vi "Get DAQmx Channels Status.vi"(0 "DAQmx task":refnum<k21>, 9 "status info in":variant, 11 "error in":errorcluster) -> (4 "DAQmx task":refnum<k21>, 6 "channel errors":bool, 10 "status info out":variant, 15 "error out":errorcluster)   [LabVIEW 2024, in "DSA_CFG_ACQ.lvlib"]
uses:
  DSA_CFG_ACQ.lvlib
  <resource>/objmgr/daqmx.rc
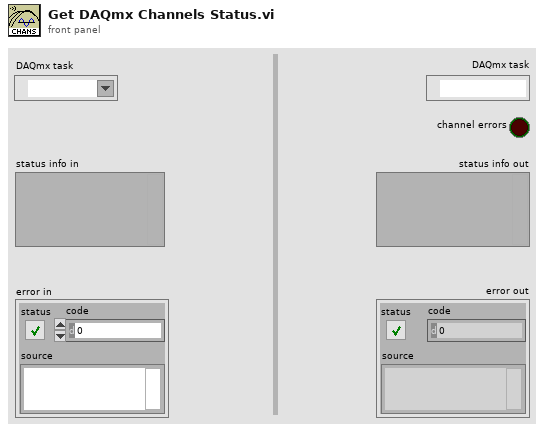
[diagram p1: front panel]
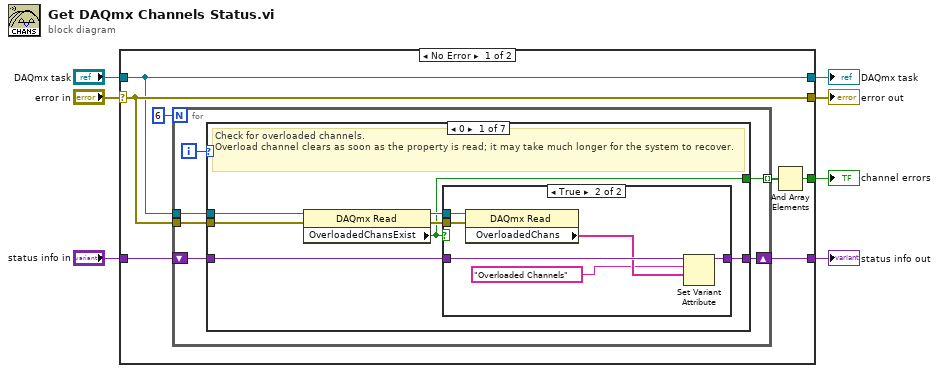
[diagram p0: block diagram]
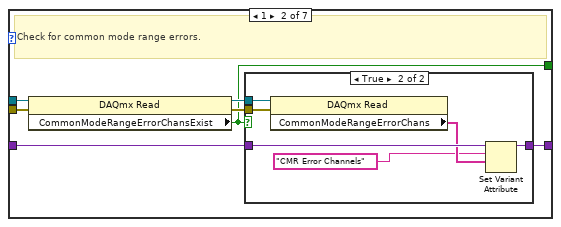
[diagram p3: hidden frame]
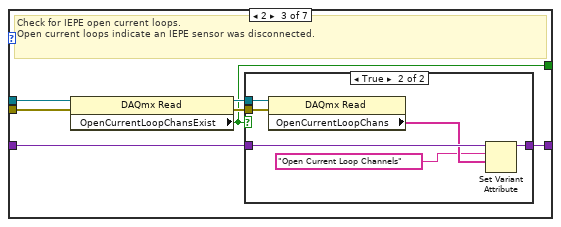
[diagram p5: hidden frame]
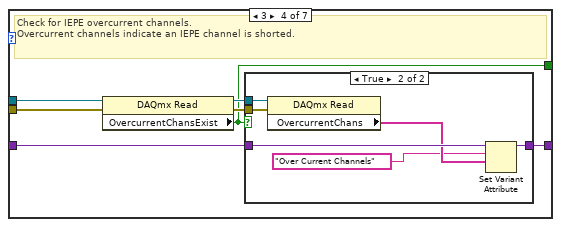
[diagram p7: hidden frame]
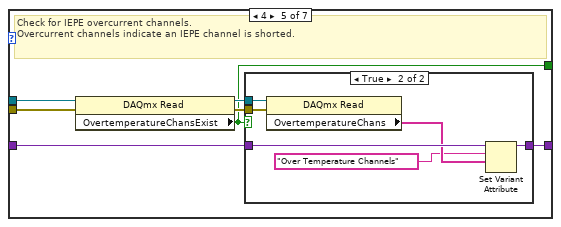
[diagram p9: hidden frame]
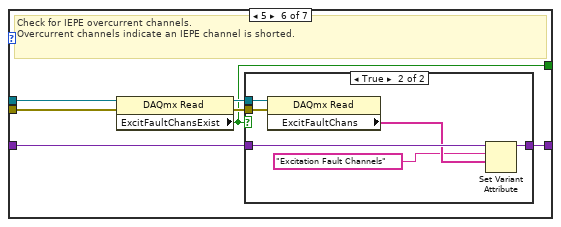
[diagram p11: hidden frame]
diagram:
  n1 = case shown="No Error" "error in" {
    selector: "error in" -> [w11 w107]
    tunnel: "DAQmx task" -> [w10 w108]
    tunnel: [w10 w108] -> w6
    tunnel: [w14 w106] -> w5
    tunnel: [w11 w107] -> w4
    tunnel: "status info in" -> [w12 w106]
    tunnel: [w8 _] -> w1
    frame No Error {
      n2 = for {
        N: 6 -> [_]
        tunnel: w11 -> [w17]
        shift-right: [w19] -> w14
        shift-left: w12 -> [w18]
        tunnel: w10 -> [w20]
        tunnel: [w15] -> w9 mode=indexing
        i -> [w16]
        n3 = case shown="0" w16 {
          tunnel: w20 -> [w26 w39 w53 w67 w81 w95 _]
          tunnel: [w25 w37 w50 w64 w78 w92 w105] -> w19
          tunnel: w18 -> [w24 w36 w51 w65 w79 w93 w105]
          tunnel: w17 -> [w22 w38 w52 w66 w80 w94 _]
          tunnel: [w21 w35 w49 w63 w77 w91 _] -> w15
          frame 0 {
            # "Check for overloaded channels.\nOverload channel clears as soon as the property is read; it may take much longer for the system to recover."
            n4 = property class="DAQmx Read"(reference=w26, error in=w22) -> (reference out=w27:refnum<k21>, error out=w23:errorcluster, "OverloadedChansExist"=w21:bool)
            n5 = case shown="True" w21 {
              tunnel: w27 -> [_ w34]
              tunnel: w23 -> [_ w33]
              tunnel: w24 -> [w28 w32]
              tunnel: [w28 w31] -> w25
              frame False {
              }
              frame True {
                n6 = property class="DAQmx Read"(reference=w34, error in=w33) -> ("OverloadedChans"=w30:string[])  [unwired: 2 out]
                n7 = Set Variant Attribute(Variant=w32, name="Overloaded Channels", value=w30) -> (Variant out=w31:variant)  [unwired: 1 in, 2 out]
              }
            }
          }
          frame 1 {
            # "Check for common mode range errors."
            n8 = property class="DAQmx Read"(reference=w39, error in=w38) -> (reference out=w40:refnum<k21>, error out=w41:errorcluster, "CommonModeRangeErrorChansExist"=w35:bool)
            n9 = case shown="True" w35 {
              tunnel: w40 -> [_ w48]
              tunnel: w36 -> [w42 w47]
              tunnel: [w42 w46] -> w37
              tunnel: w41 -> [_ w43]
              frame False {
              }
              frame True {
                n10 = property class="DAQmx Read"(reference=w48, error in=w43) -> ("CommonModeRangeErrorChans"=w45:string[])  [unwired: 2 out]
                n11 = Set Variant Attribute(Variant=w47, name="CMR Error Channels", value=w45) -> (Variant out=w46:variant)  [unwired: 1 in, 2 out]
              }
            }
          }
          frame 2 {
            # "Check for IEPE open current loops.\nOpen current loops indicate an IEPE sensor was disconnected."
            n12 = property class="DAQmx Read"(reference=w53, error in=w52) -> (reference out=w54:refnum<k21>, error out=w55:errorcluster, "OpenCurrentLoopChansExist"=w49:bool)
            n13 = case shown="True" w49 {
              tunnel: w54 -> [_ w62]
              tunnel: w51 -> [w56 w61]
              tunnel: [w56 w60] -> w50
              tunnel: w55 -> [_ w58]
              frame False {
              }
              frame True {
                n14 = property class="DAQmx Read"(reference=w62, error in=w58) -> ("OpenCurrentLoopChans"=w59:string[])  [unwired: 2 out]
                n15 = Set Variant Attribute(Variant=w61, name="Open Current Loop Channels", value=w59) -> (Variant out=w60:variant)  [unwired: 1 in, 2 out]
              }
            }
          }
          frame 3 {
            # "Check for IEPE overcurrent channels.\nOvercurrent channels indicate an IEPE channel is shorted."
            n16 = property class="DAQmx Read"(reference=w67, error in=w66) -> (reference out=w69:refnum<k21>, error out=w68:errorcluster, "OvercurrentChansExist"=w63:bool)
            n17 = case shown="True" w63 {
              tunnel: w69 -> [_ w76]
              tunnel: w65 -> [w70 w75]
              tunnel: [w70 w74] -> w64
              tunnel: w68 -> [_ w72]
              frame False {
              }
              frame True {
                n18 = property class="DAQmx Read"(reference=w76, error in=w72) -> ("OvercurrentChans"=w73:string[])  [unwired: 2 out]
                n19 = Set Variant Attribute(Variant=w75, name="Over Current Channels", value=w73) -> (Variant out=w74:variant)  [unwired: 1 in, 2 out]
              }
            }
          }
          frame 4 {
            # "Check for IEPE overcurrent channels.\nOvercurrent channels indicate an IEPE channel is shorted."
            n20 = property class="DAQmx Read"(reference=w81, error in=w80) -> (reference out=w83:refnum<k21>, error out=w82:errorcluster, "OvertemperatureChansExist"=w77:bool)
            n21 = case shown="True" w77 {
              tunnel: w83 -> [_ w90]
              tunnel: w79 -> [w84 w89]
              tunnel: [w84 w88] -> w78
              tunnel: w82 -> [_ w86]
              frame False {
              }
              frame True {
                n22 = property class="DAQmx Read"(reference=w90, error in=w86) -> ("OvertemperatureChans"=w87:string[])  [unwired: 2 out]
                n23 = Set Variant Attribute(Variant=w89, name="Over Temperature Channels", value=w87) -> (Variant out=w88:variant)  [unwired: 1 in, 2 out]
              }
            }
          }
          frame 5 {
            # "Check for IEPE overcurrent channels.\nOvercurrent channels indicate an IEPE channel is shorted."
            n24 = property class="DAQmx Read"(reference=w95, error in=w94) -> (reference out=w97:refnum<k21>, error out=w96:errorcluster, "ExcitFaultChansExist"=w91:bool)
            n25 = case shown="True" w91 {
              tunnel: w97 -> [_ w104]
              tunnel: w93 -> [w98 w103]
              tunnel: [w98 w102] -> w92
              tunnel: w96 -> [_ w100]
              frame False {
              }
              frame True {
                n26 = property class="DAQmx Read"(reference=w104, error in=w100) -> ("ExcitFaultChans"=w101:string[])  [unwired: 2 out]
                n27 = Set Variant Attribute(Variant=w103, name="Excitation Fault Channels", value=w101) -> (Variant out=w102:variant)  [unwired: 1 in, 2 out]
              }
            }
          }
          frame Default {
            # "You should never get to the case with value wired to N value of For Loop because iteration count starts at zero and increments up to N-1."
          }
        }
      }
      n28 = And Array Elements(Boolean array=w9) -> (logical AND=w8:bool)
    }
    frame Error {
    }
  }
  "status info out" <- w5
  "error out" <- w4
  "DAQmx task" <- w6
  "channel errors" <- w1
